vi "查询启动项.vi"(8 "error in (no error)":errorcluster caption="错误输入（无错误）") -> (0 "error out":errorcluster caption="错误输出", 2 "values":string[](array[string]) caption="值", 3 "包含启动项":bool)   [LabVIEW 2016]
uses:
  <vilib>/registry/registry.llb/Registry RtKey.ctl
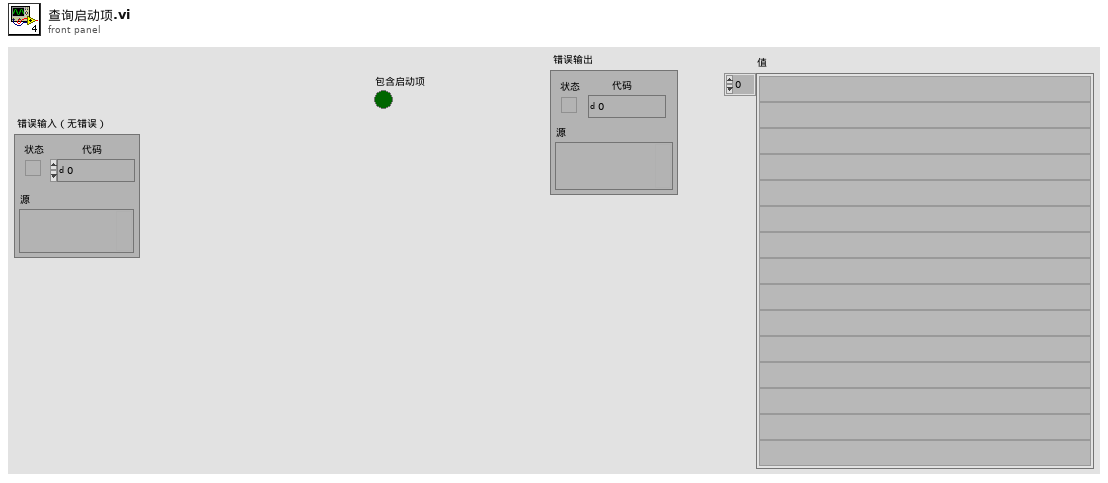
[diagram p1: front panel]
types:
  T1 = typedef "Registry RtKey.ctl" = enum32{"HKEY_CLASSES_ROOT", "HKEY_CURRENT_USER", "HKEY_LOCAL_MACHINE", "HKEY_USERS", "HKEY_PERFORMANCE_DATA", "HKEY_CURRENT_CONFIG", "HKEY_DYN_DATA"}
  T2 = typedef "Registry refnum.ctl" = refnum<k1>
  T3 = cluster{"numValues":i32, "maxValueNameLen":i32, "maxValueDataLen":i32}
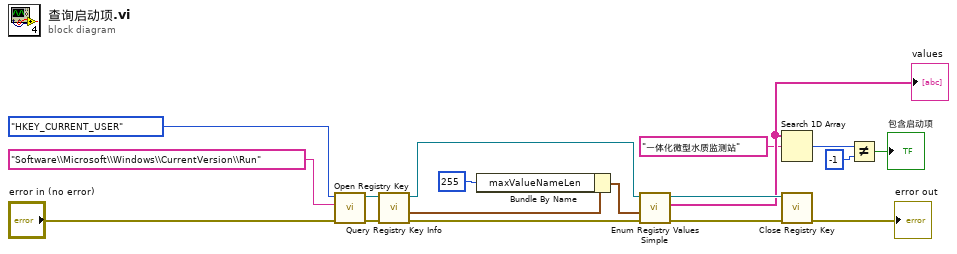
[diagram p0: block diagram]
diagram:
  n1 = call <vilib>:"Open Registry Key.vi"("error in (no error)"="error in (no error)", "subkey"="Software\\Microsoft\\Windows\\CurrentVersion\\Run", "root key (HKEY_LOCAL_MACHINE)"=Registry_RtKey."HKEY_CURRENT_USER") -> ("error out"=w14:errorcluster, "refnum out"=w15:T2)  [unwired: 7 in]
  n2 = call <vilib>:"Query Registry Key Info.vi"("error in (no error)"=w14, "refnum"=w15) -> ("error out"=w11:errorcluster, "value info"=w12:T3, "refnum out"=w13:T2)  [unwired: 5 in, 2 out]
  n3 = Bundle By Name(cluster=w12, "maxValueNameLen"=255) -> (w2:T3)
  n4 = call <vilib>:"Enum Registry Values Simple.vi"("error in (no error)"=w11, "value info"=w2, "refnum"=w13) -> ("error out"=w9:errorcluster, "values"=w8:string[], "refnum out"=w10:T2)  [unwired: 3 in, 3 out]
  "values" <- w8
  n5 = Search 1D Array(1D array=w8, element="一体化微型水质监测站" ("元素")) -> (index of element=w7:i32)  [unwired: 1 in]
  n6 = call <vilib>:"Close Registry Key.vi"("error in (no error)"=w9, "refnum"=w10) -> ("error out"=→"error out":errorcluster)  [unwired: 5 in]
  n7 = Not Equal?(x=w7, y=-1) -> (x != y?=→"包含启动项":bool)
